vi "Sample.vi"(8 "error in (no error)":errorcluster, 10 "Sample Dimensions":T1, 11 "Cubes in":refnum<class "Cubes.lvclass">) -> (0 "error out":errorcluster, 2 "N Cubes":i64, 3 "Cubes out":refnum<class "Cubes.lvclass">)   [LabVIEW 2019, in "22.lvlib" / "Cubes.lvclass"]
uses:
  Cubes.lvclass
  Cube/Cube.lvclass
  Cubes.lvclass/Cubes.ctl
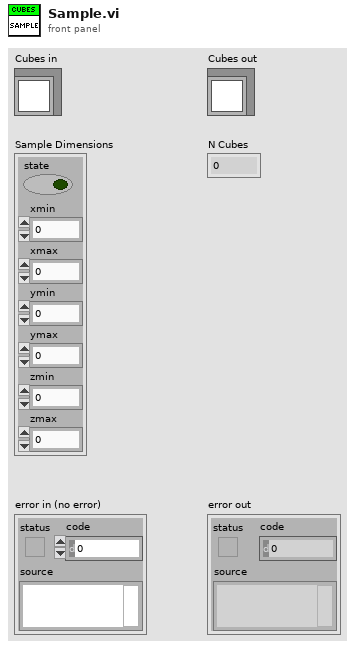
[diagram p1: front panel]
types:
  T1 = cluster{"state":bool, "xmin":i64, "xmax":i64, "ymin":i64, "ymax":i64, "zmin":i64, "zmax":i64}
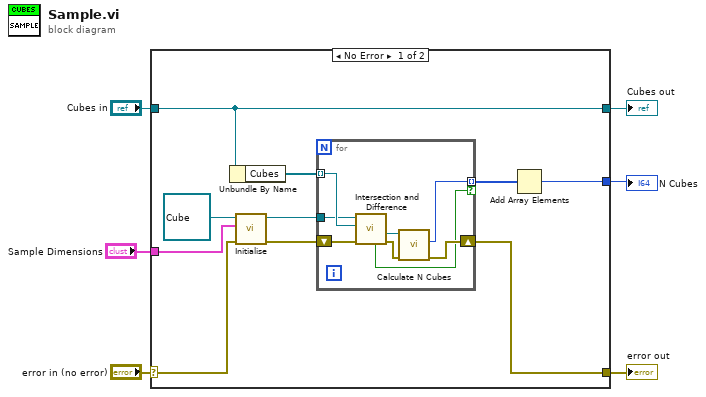
[diagram p0: block diagram]
diagram:
  n1 = case shown="No Error" "error in (no error)" {
    selector: "error in (no error)" -> [w10 w26]
    tunnel: [w14 w26] -> w5
    tunnel: [w16 w25] -> w3
    tunnel: "Cubes in" -> [w16 w25]
    tunnel: [w12 _] -> w2
    tunnel: "Sample Dimensions" -> [w7 _]
    frame No Error {
      n2 = Unbundle By Name(w16) -> ("Cubes"=w15:refnum<class "Cube.lvclass">[])
      n3 = call-dynamic "Initialise.vi"("error in (no error)"=w10, "Init"=w7, "Cube in"=refnum<class "Cube.lvclass"> refnum ("22.lvlib:Cube.lvclass")) -> ("error out"=w9:errorcluster, "Cube out"=w8:refnum<class "Cube.lvclass">)  [unwired: 7 in]
      n4 = for {
        tunnel: w15 -> [w22] mode=indexing
        tunnel: [w24] -> w13 mode=indexing if=w17
        shift-right: [w23] -> w14
        shift-left: w9 -> [w19]
        tunnel: w8 -> [w21]
        n5 = call-dynamic "Intersection and Difference.vi"("error in (no error)"=w19, "Cube A"=w22, "Cube B in"=w21) -> ("error out"=w18:errorcluster, "Intersection"=w20:refnum<class "Cube.lvclass">, "Intersection Found?"=w17:bool)  [unwired: 4 in, 2 out]
        n6 = call-dynamic "Calculate N Cubes.vi"("error in (no error)"=w18, "Cube in"=w20) -> ("error out"=w23:errorcluster, "N Cubes"=w24:i64)  [unwired: 7 in, 1 out]
      }
      n7 = Add Array Elements(numeric array=w13) -> (sum=w12:i64)
    }
    frame Error {
    }
  }
  "error out" <- w5
  "Cubes out" <- w3
  "N Cubes" <- w2
